vi "AssessRectangle.vi"(0 "Coords In 1":T3, 2 "Coords In 2":T3, 8 "Tool":T1) -> (15 "Rectangle":T2)   [LabVIEW 2020]
uses:
  <vilib>/Utility/miscctls.llb/LVPoint32TypeDef.ctl
  Controls/Circle.ctl
  Controls/Dropper.ctl
  Controls/FCircle.ctl
  Controls/Fill.ctl
  Controls/FRect.ctl
  Controls/Line.ctl
  Controls/Move.ctl
  Controls/Pen.ctl
  Controls/IERect.ctl
  Controls/Rubber.ctl
  Controls/Selection.ctl
  Controls/Text.ctl
  Controls/Tools.ctl
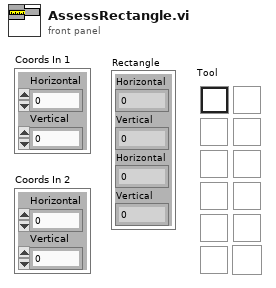
[diagram p1: front panel]
types:
  T1 = typedef "Tools.ctl" = enum32{"Pencil", "Line", "Dropper", "Fill", "Rectangle", "Filled Rectangle", "Ellipse", "Filled Ellipse", "Eraser", "Text", "Select", "Move"}
  T2 = cluster{"Horizontal":i32, "Vertical":i32, "Horizontal":i32, "Vertical":i32}
  T3 = typedef "LVPoint32TypeDef.ctl" = cluster{"Horizontal":i32, "Vertical":i32}
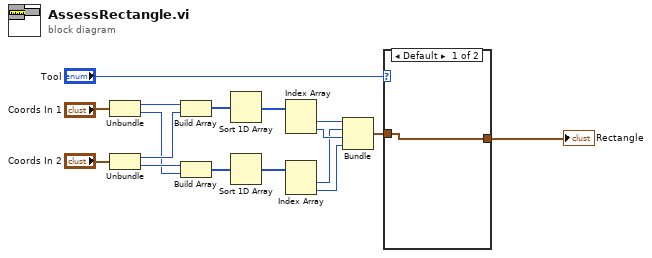
[diagram p0: block diagram]
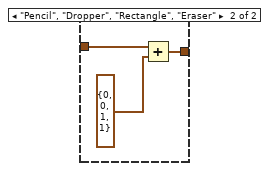
[diagram p2: hidden frame]
diagram:
  n1 = Unbundle("Coords In 1") -> ("Horizontal"=w15:i32, "Vertical"=w12:i32)
  n2 = Unbundle("Coords In 2") -> ("Horizontal"=w14:i32, "Vertical"=w13:i32)
  n3 = Build Array(w15, w14) -> (w11:i32[])
  n4 = Build Array(w13, w12) -> (w10:i32[])
  n5 = Sort 1D Array(array=w11) -> (sorted array=w9:i32[])
  n6 = Sort 1D Array(array=w10) -> (sorted array=w8:i32[])
  n7 = Index Array(array=w9) -> (element #1=w7:i32, element #2=w6:i32)  [unwired: 2 in]
  n8 = Index Array(array=w8) -> (element #1=w5:i32, element #2=w4:i32)  [unwired: 2 in]
  n9 = Bundle("Horizontal"=w7, "Vertical"=w5, "Horizontal"=w6, "Vertical"=w4) -> (w2:T2)  [unwired: 1 out]
  n10 = case shown="Default" "Tool" {
    tunnel: w2 -> [w18 w21]
    tunnel: [w18 w19] -> w1
    frame Default {
    }
    frame "Pencil", "Dropper", "Rectangle", "Eraser" {
      n11 = Add(x=w21, y=T2 {"Horizontal"=0, "Vertical"=0, "Horizontal"=1, "Vertical"=1} ("output cluster")) -> (x+y=w19:T2)
    }
  }
  "Rectangle" <- w1
